vi "Stage_handle_ae.vi"(9 "VISA In":refnum<visa-resource-name>, 10 "StageID":string, 11 "Enum":enum16{"WRITE", "READ"}(ring)) -> (1 "Visa Out":refnum<visa-resource-name>)   [LabVIEW 2014]
panel:
  in  "Stage handles":T1
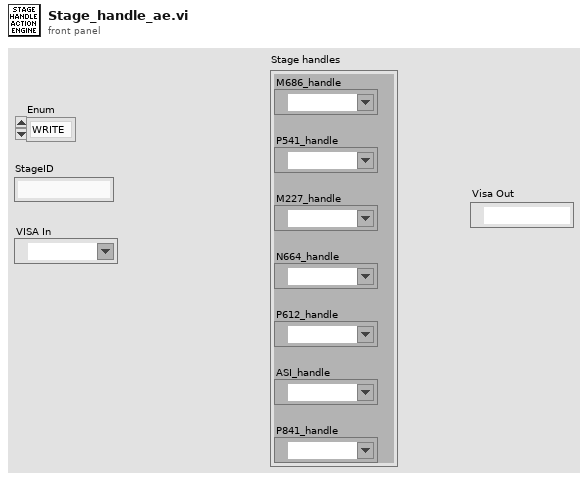
[diagram p1: front panel]
types:
  T1 = cluster{"M686_handle":refnum<visa-resource-name>, "P541_handle":refnum<visa-resource-name>, "M227_handle":refnum<visa-resource-name>, "N664_handle":refnum<visa-resource-name>, "P612_handle":refnum<visa-resource-name>, "ASI_handle":refnum<visa-resource-name>, "P841_handle":refnum<visa-resource-name>}
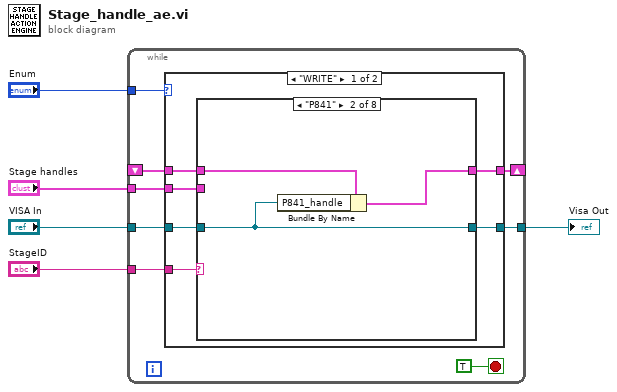
[diagram p0: block diagram]
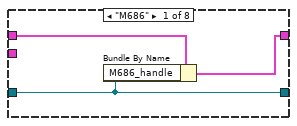
[diagram p2: hidden frame]
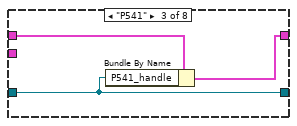
[diagram p3: hidden frame]
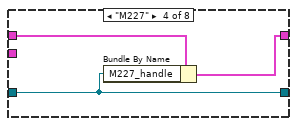
[diagram p4: hidden frame]
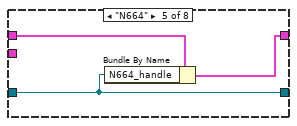
[diagram p5: hidden frame]
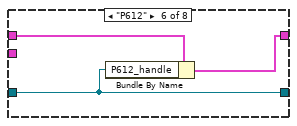
[diagram p6: hidden frame]
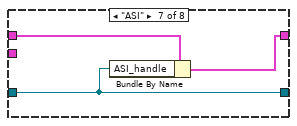
[diagram p7: hidden frame]
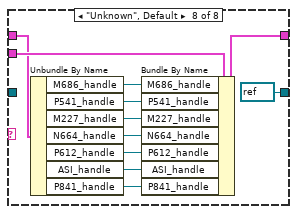
[diagram p8: hidden frame]
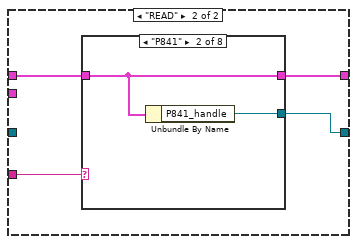
[diagram p9: hidden frame]
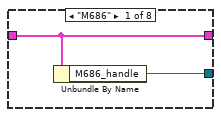
[diagram p10: hidden frame]
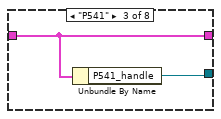
[diagram p11: hidden frame]
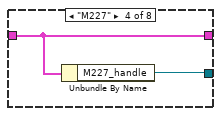
[diagram p12: hidden frame]
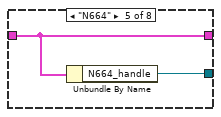
[diagram p13: hidden frame]
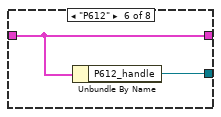
[diagram p14: hidden frame]
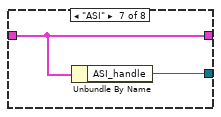
[diagram p15: hidden frame]
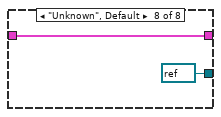
[diagram p16: hidden frame]
diagram:
  n1 = while {
    tunnel: "StageID" -> [w9]
    tunnel: "Enum" -> [w12]
    shift-right: [w11] -> _
    shift-left: _ -> [w10]
    tunnel: "Stage handles" -> [w8]
    tunnel: "VISA In" -> [w7]
    tunnel: [w6] -> w1
    stop <- TRUE stop-if-true
    n2 = case shown="\"WRITE\"" w12 {
      tunnel: [w19 w55] -> w11
      tunnel: w10 -> [w14 w53]
      tunnel: w9 -> [w18 w54]
      tunnel: w8 -> [w17 _]
      tunnel: w7 -> [w16 _]
      tunnel: [w15 w52] -> w6
      frame "WRITE" {
        n3 = case shown="\"P841\"" w18 {
          tunnel: [w22 w23 w28 w31 w34 w37 w40 w50] -> w19
          tunnel: w17 -> [_ _ _ _ _ _ _ w51]
          tunnel: w16 -> [w21 w24 w27 w30 w33 w36 w39 _]
          tunnel: [w21 w24 w27 w30 w33 w36 w39 refnum<visa-resource-name> refnum ("VISA In")] -> w15
          tunnel: w14 -> [w20 w25 w26 w29 w32 w35 w38 w49]
          frame "M686" {
            n4 = Bundle By Name(cluster=w20, "M686_handle"=w21) -> (w22:T1)
          }
          frame "P841" {
            n5 = Bundle By Name(cluster=w25, "P841_handle"=w24) -> (w23:T1)
          }
          frame "P541" {
            n6 = Bundle By Name(cluster=w26, "P541_handle"=w27) -> (w28:T1)
          }
          frame "M227" {
            n7 = Bundle By Name(cluster=w29, "M227_handle"=w30) -> (w31:T1)
          }
          frame "N664" {
            n8 = Bundle By Name(cluster=w32, "N664_handle"=w33) -> (w34:T1)
          }
          frame "P612" {
            n9 = Bundle By Name(cluster=w35, "P612_handle"=w36) -> (w37:T1)
          }
          frame "ASI" {
            n10 = Bundle By Name(cluster=w38, "ASI_handle"=w39) -> (w40:T1)
          }
          frame "Unknown", Default {
            n11 = Unbundle By Name(w49) -> ("M686_handle"=w48:refnum<visa-resource-name>, "P541_handle"=w47:refnum<visa-resource-name>, "M227_handle"=w46:refnum<visa-resource-name>, "N664_handle"=w45:refnum<visa-resource-name>, "P612_handle"=w44:refnum<visa-resource-name>, "ASI_handle"=w43:refnum<visa-resource-name>, "P841_handle"=w41:refnum<visa-resource-name>)
            n12 = Bundle By Name(cluster=w51, "M686_handle"=w48, "P541_handle"=w47, "M227_handle"=w46, "N664_handle"=w45, "P612_handle"=w44, "ASI_handle"=w43, "P841_handle"=w41) -> (w50:T1)
          }
        }
      }
      frame "READ" {
        n13 = case shown="\"P841\"" w54 {
          tunnel: [w57 w59 w61 w63 w65 w67 w69 w71] -> w55
          tunnel: w53 -> [w57 w59 w61 w63 w65 w67 w69 w71]
          tunnel: [w56 w58 w60 w62 w64 w66 w68 refnum<visa-resource-name> refnum ("ASI_handle")] -> w52
          frame "M686" {
            n14 = Unbundle By Name(w57) -> ("M686_handle"=w56:refnum<visa-resource-name>)
          }
          frame "P841" {
            n15 = Unbundle By Name(w59) -> ("P841_handle"=w58:refnum<visa-resource-name>)
          }
          frame "P541" {
            n16 = Unbundle By Name(w61) -> ("P541_handle"=w60:refnum<visa-resource-name>)
          }
          frame "M227" {
            n17 = Unbundle By Name(w63) -> ("M227_handle"=w62:refnum<visa-resource-name>)
          }
          frame "N664" {
            n18 = Unbundle By Name(w65) -> ("N664_handle"=w64:refnum<visa-resource-name>)
          }
          frame "P612" {
            n19 = Unbundle By Name(w67) -> ("P612_handle"=w66:refnum<visa-resource-name>)
          }
          frame "ASI" {
            n20 = Unbundle By Name(w69) -> ("ASI_handle"=w68:refnum<visa-resource-name>)
          }
          frame "Unknown", Default {
          }
        }
      }
    }
  }
  "Visa Out" <- w1
